vi "add_head.vi"(8 "error in (no error)":errorcluster, 10 "data":dbl, 11 "DoublyLinkedList in":refnum<class "DoublyLinkedList.lvclass">) -> (0 "error out":errorcluster, 3 "DoublyLinkedList out":refnum<class "DoublyLinkedList.lvclass">)   [LabVIEW 2021, in "DoublyLinkedList.lvclass"]
uses:
  DoublyLinkedList.lvclass
  DoublyLinkedList.lvclass/DoublyLinkedList.ctl
  Iterator/Iterator.lvclass
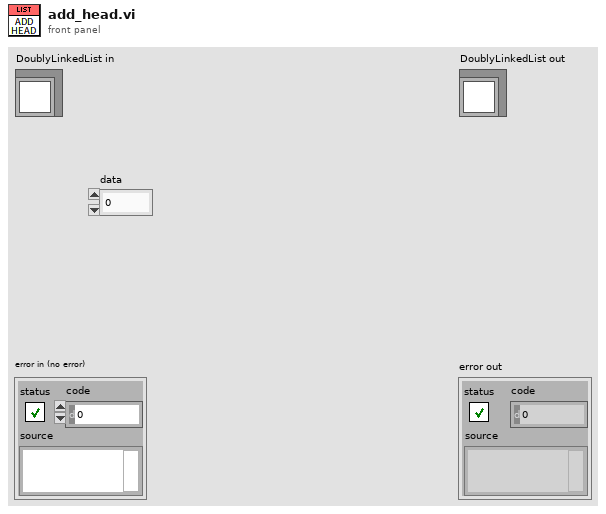
[diagram p1: front panel]
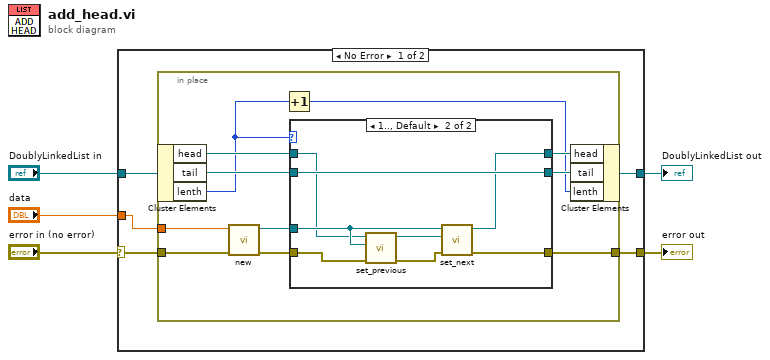
[diagram p0: block diagram]
diagram:
  n1 = case shown="No Error" "error in (no error)" {
    selector: "error in (no error)" -> [w8 w33]
    tunnel: [w7 w33] -> w4
    tunnel: [w6 w32] -> w2
    tunnel: "DoublyLinkedList in" -> [w10 w32]
    tunnel: "data" -> [w9 _]
    frame No Error {
      n2 = in-place {
        in-place-border: w9 -> [w18]
        in-place-border: w8 -> [w19]
        in-place-border: [w15] -> w7
        n3 = in-place-cluster #1(w10) -> ("head"=w21:refnum<class "Iterator.lvclass">, "tail"=w20:refnum<class "Iterator.lvclass">, "lenth"=w14:u32)
        n4 = call "new.vi"("error in (no error)"=w19, "data"=w18) -> ("error out"=w11:errorcluster, "Iterator out"=w12:refnum<class "Iterator.lvclass">)  [unwired: 8 in]
        n5 = Increment(x=w14) -> (x+1=w13:u32)
        n6 = case shown="1.., Default" w14 {
          tunnel: [w23 w31] -> w16
          tunnel: w21 -> [_ w26]
          tunnel: w20 -> [_ w31]
          tunnel: w12 -> [w23 w28]
          tunnel: [w23 w30] -> w17
          tunnel: w11 -> [w22 w24]
          tunnel: [w22 w29] -> w15
          frame 0 {
          }
          frame 1.., Default {
            n7 = call-dynamic "set_previous.vi"("error in (no error)"=w24, "previous"=w28, "Iterator in"=w26) -> ("error out"=w27:errorcluster, "Iterator out"=w25:refnum<class "Iterator.lvclass">)  [unwired: 7 in]
            n8 = call-dynamic "set_next.vi"("error in (no error)"=w27, "next"=w25, "Iterator in"=w28) -> ("error out"=w29:errorcluster, "Iterator out"=w30:refnum<class "Iterator.lvclass">)  [unwired: 7 in]
          }
        }
        n9 = in-place-cluster #1("head"=w17, "tail"=w16, "lenth"=w13) -> (w6:refnum<class "DoublyLinkedList.lvclass">)
      }
    }
    frame Error {
    }
  }
  "error out" <- w4
  "DoublyLinkedList out" <- w2
